vi "Numeric Integration.vi"   [LabVIEW 2017, in "NI_AALPro.lvlib"]
doc: "Performs numeric integration on the <B>Input Array</B> using one of four popular numeric integration methods. \n\nWire data to the <B>Input Array</B> input to determine the polymorphic instance to use or manually select the instance."
uses:
  <vilib>/Analysis/NI_AALPro.lvlib
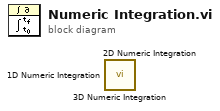
[diagram p0: block diagram]
diagram:
  n1 = call <vilib>:"3D Numeric Integration.vi"() -> ()  [unwired: 3 in, 2 out]
  n2 = call <vilib>:"2D Numeric Integration.vi"() -> ()  [unwired: 3 in, 2 out]
  n3 = call <vilib>:"1D Numeric Integration.vi"() -> ()  [unwired: 3 in, 2 out]
